vi "subVI_CONEX_getStatus.vi"(0 "CONEX Cluster":T1, 3 "Error IN":errorcluster) -> (6 "CONEX Cluster out":T1, 9 "error out":errorcluster)   [LabVIEW 2010]
panel:
  out "colors":u32[](array[numeric])
  out "Action names":string[](array[string])
  out "Controller state descriptions":string[](array[string])
  out "Positioner error descriptions":string[](array[string])
  out "appended array":bool[][][](array[boolean])
  out "Positioner Error boolean arrays":bool[](array[boolean])
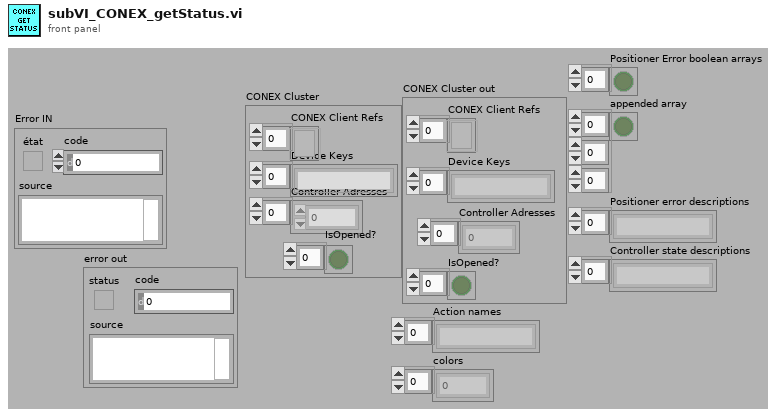
[diagram p1: front panel]
types:
  T1 = cluster{"CONEX Client Refs":refnum<k24>[], "Device Keys":string[], "Controller Adresses":i32[], "IsOpened?":bool[]}
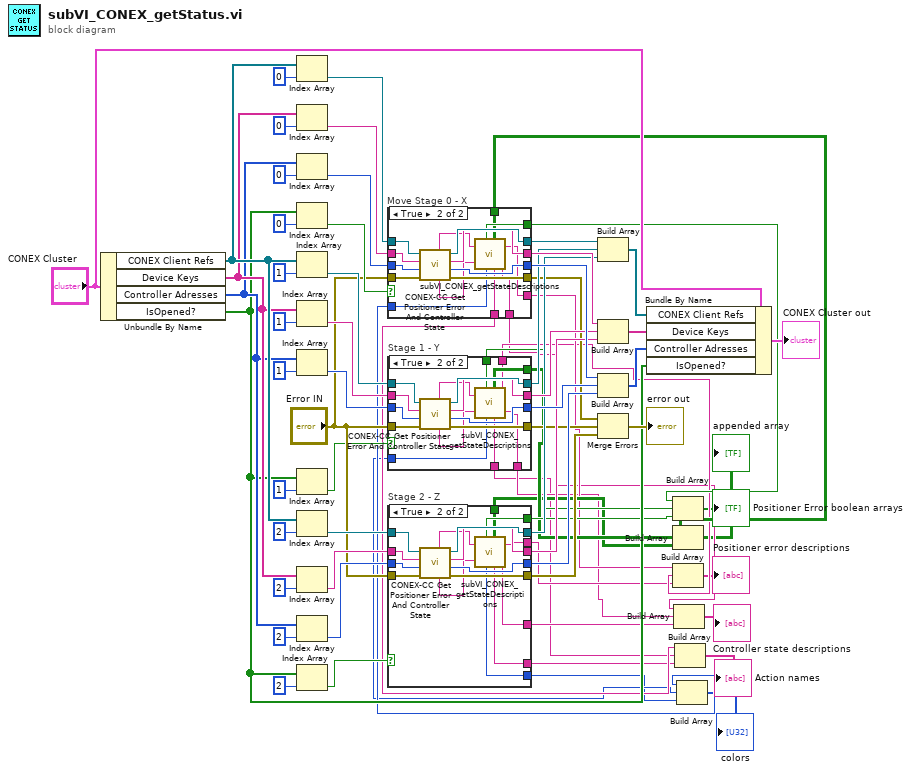
[diagram p0: block diagram]
diagram:
  n1 = Unbundle By Name("CONEX Cluster") -> ("CONEX Client Refs"=w68:refnum<k24>[], "Device Keys"=w63:string[], "Controller Adresses"=w58:i32[], "IsOpened?"=w27:bool[])
  n2 = Index Array(array=w68, index=0) -> (element=w67:refnum<k24>)
  n3 = Index Array(array=w63, index=0) -> (element=w62:string)
  n4 = Index Array(array=w58, index=0) -> (element=w57:i32)
  n5 = Index Array(array=w27, index=0) -> (element=w48:bool)
  n6 = Index Array(array=w68, index=1) -> (element=w46:refnum<k24>)
  n7 = Index Array(array=w63, index=1) -> (element=w44:string)
  n8 = Index Array(array=w58, index=1) -> (element=w41:i32)
  n9 = Index Array(array=w27, index=1) -> (element=w25:bool)
  n10 = Index Array(array=w68, index=2) -> (element=w45:refnum<k24>)
  n11 = Index Array(array=w63, index=2) -> (element=w43:string)
  n12 = Index Array(array=w58, index=2) -> (element=w42:i32)
  n13 = Index Array(array=w27, index=2) -> (element=w28:bool)
  n14 = case "Move Stage 0 - X" shown="True" w48 {
    tunnel: w67 -> [w72 w91]
    tunnel: w62 -> [w73 w90]
    tunnel: w57 -> [w74 w89]
    tunnel: "Error IN" -> [w75 w88]
    tunnel: [w72 w87] -> w56
    tunnel: [w73 w86] -> w55
    tunnel: [w74 w85] -> w54
    tunnel: [w75 w84] -> w30
    tunnel: [_ w81] -> w24
    tunnel: [_ w80] -> w21
    tunnel: [_ w79] -> w18
    tunnel: [_ w78] -> w15
    tunnel: [_ w77] -> w12
    tunnel: [_ w76] -> w9
    frame False {
    }
    frame True {
      n15 = call <userlib>:"CONEX-CC Get Positioner Error And Controller State.vi"("CONEX Client Ref IN"=w91, "deviceKey"=w90, "Address IN"=w89, "Error IN"=w88) -> ("Positioner error"=w83:string, "Controller state"=w82:string, "CONEX Client Ref OUT"=w87:refnum<k24>, "deviceKey OUT"=w86:string, "Address OUT"=w85:i32, "Error OUT"=w84:errorcluster)
      n16 = call "subVI_CONEX_getStateDescriptions.vi"("Controller state"=w82, "Positioner error"=w83) -> ("Color"=w76:u32, "Action name"=w77:string, "Controller state description"=w78:string, "IsReady?"=w81:bool, "Positioner error boolean array"=w80:bool[][], "Positioner error description"=w79:string)
    }
  }
  n17 = case "Stage 1 - Y" shown="True" w25 {
    tunnel: w46 -> [w92 w111]
    tunnel: w44 -> [w93 w110]
    tunnel: w41 -> [w94 w109]
    tunnel: "Error IN" -> [w95 w108]
    tunnel: [w92 w107] -> w34
    tunnel: [w93 w106] -> w37
    tunnel: [w94 w105] -> w38
    tunnel: [w95 w104] -> w33
    tunnel: [_ w101] -> w23
    tunnel: [_ w100] -> w20
    tunnel: [_ w99] -> w17
    tunnel: [_ w98] -> w14
    tunnel: [_ w97] -> w11
    tunnel: [_ w96] -> w8
    frame False {
    }
    frame True {
      n18 = call <userlib>:"CONEX-CC Get Positioner Error And Controller State.vi"("CONEX Client Ref IN"=w111, "deviceKey"=w110, "Address IN"=w109, "Error IN"=w108) -> ("Positioner error"=w102:string, "Controller state"=w103:string, "CONEX Client Ref OUT"=w107:refnum<k24>, "deviceKey OUT"=w106:string, "Address OUT"=w105:i32, "Error OUT"=w104:errorcluster)
      n19 = call "subVI_CONEX_getStateDescriptions.vi"("Controller state"=w103, "Positioner error"=w102) -> ("Color"=w96:u32, "Action name"=w97:string, "Controller state description"=w98:string, "IsReady?"=w101:bool, "Positioner error boolean array"=w100:bool[][], "Positioner error description"=w99:string)
    }
  }
  n20 = case "Stage 2 - Z" shown="True" w28 {
    tunnel: w45 -> [w112 w131]
    tunnel: w43 -> [w113 w130]
    tunnel: w42 -> [w114 w129]
    tunnel: "Error IN" -> [w115 w128]
    tunnel: [w112 w127] -> w35
    tunnel: [w113 w126] -> w36
    tunnel: [w114 w125] -> w39
    tunnel: [w115 w124] -> w32
    tunnel: [_ w121] -> w22
    tunnel: [_ w120] -> w19
    tunnel: [_ w119] -> w16
    tunnel: [_ w118] -> w13
    tunnel: [_ w117] -> w10
    tunnel: [_ w116] -> w7
    frame False {
    }
    frame True {
      n21 = call <userlib>:"CONEX-CC Get Positioner Error And Controller State.vi"("CONEX Client Ref IN"=w131, "deviceKey"=w130, "Address IN"=w129, "Error IN"=w128) -> ("Positioner error"=w122:string, "Controller state"=w123:string, "CONEX Client Ref OUT"=w127:refnum<k24>, "deviceKey OUT"=w126:string, "Address OUT"=w125:i32, "Error OUT"=w124:errorcluster)
      n22 = call "subVI_CONEX_getStateDescriptions.vi"("Controller state"=w123, "Positioner error"=w122) -> ("Color"=w116:u32, "Action name"=w117:string, "Controller state description"=w118:string, "IsReady?"=w121:bool, "Positioner error boolean array"=w120:bool[][], "Positioner error description"=w119:string)
    }
  }
  n23 = Build Array(w56, w34, w35) -> (w53:refnum<k24>[])
  n24 = Build Array(w55, w37, w36) -> (w52:string[])
  n25 = Build Array(w54, w38, w39) -> (w51:i32[])
  n26 = Merge Errors(w30, w33, w32) -> (→"error out":errorcluster)
  n27 = Bundle By Name(cluster="CONEX Cluster", "CONEX Client Refs"=w53, "Device Keys"=w52, "Controller Adresses"=w51, "IsOpened?"=w27) -> (→"CONEX Cluster out":T1)
  n28 = Build Array(w24, w23, w22) -> (→"Positioner Error boolean arrays":bool[])
  n29 = Build Array(w21, w20, w19) -> (→"appended array":bool[][][])
  n30 = Build Array(w18, w17, w16) -> (→"Positioner error descriptions":string[])
  n31 = Build Array(w15, w14, w13) -> (→"Controller state descriptions":string[])
  n32 = Build Array(w12, w11, w10) -> (→"Action names":string[])
  n33 = Build Array(w9, w8, w7) -> (→"colors":u32[])
